vi "main.vi"() -> ()   [LabVIEW 2021]
uses:
  <vilib>/Utility/error.llb/Error Cluster From Error Code.vi
  <vilib>/ErrorRing/Error Ring.xnode
  Ctls/msg.ctl
  <vilib>/MakerHub/LINX/LMH-LINX.lvlib
  <vilib>/MakerHub/LINX/Private/Type Defs/Platform.ctl
  <vilib>/MakerHub/LINX/Private/Type Defs/Interface.ctl
  <vilib>/MakerHub/LINX/Private/Device/Type Defs/TCP Config.ctl
  <vilib>/MakerHub/LINX/Private/Device/Device.lvlib
  <vilib>/MakerHub/LINX/Private/Device/Type Defs/Channels.ctl
  <vilib>/MakerHub/LINX/Private/Device/Type Defs/LINX Device Config.ctl
  <vilib>/MakerHub/LINX/Private/Type Defs/LINX Ref.ctl
  <vilib>/MakerHub/LINX/Public/Utilities/Open Serial.vi
  Global 1.vi
panel:
  in  "Buadrate":u32=8
  out "?":bool
  out "Trama Leída w/r":string
  in  "Número de bytes a leer":u8=32
  in  "Dirección Esclavo (w/r)":u8=8
  in  "Envio":string
  in  "WaR":bool
  out "?":bool
  out "?":bool
  out "Status":bool
  in  "Stop":bool
  in  "Dirección Esclavo Escritura":u8=8
  in  "Dirección Eslcavo Lectura":u8=8
  in  "Número de bytes a leer":u8=32
  out "Trama Leída":string
  in  "Data":string
  in  "Puerto COM":refnum<visa-resource-name>
  in  "Read":bool
  in  "Write":bool
  in  "error in (no error) 3":errorcluster
  out "error in (no error) 2":errorcluster
  out "Data":u8[](array[numeric])
  in  "error in (no error)":errorcluster
  # "LECTURA"
  # "ESCRITURA"
  # "CONFIGURACIÓN"
  # "ESCRITURA/LECTURA"
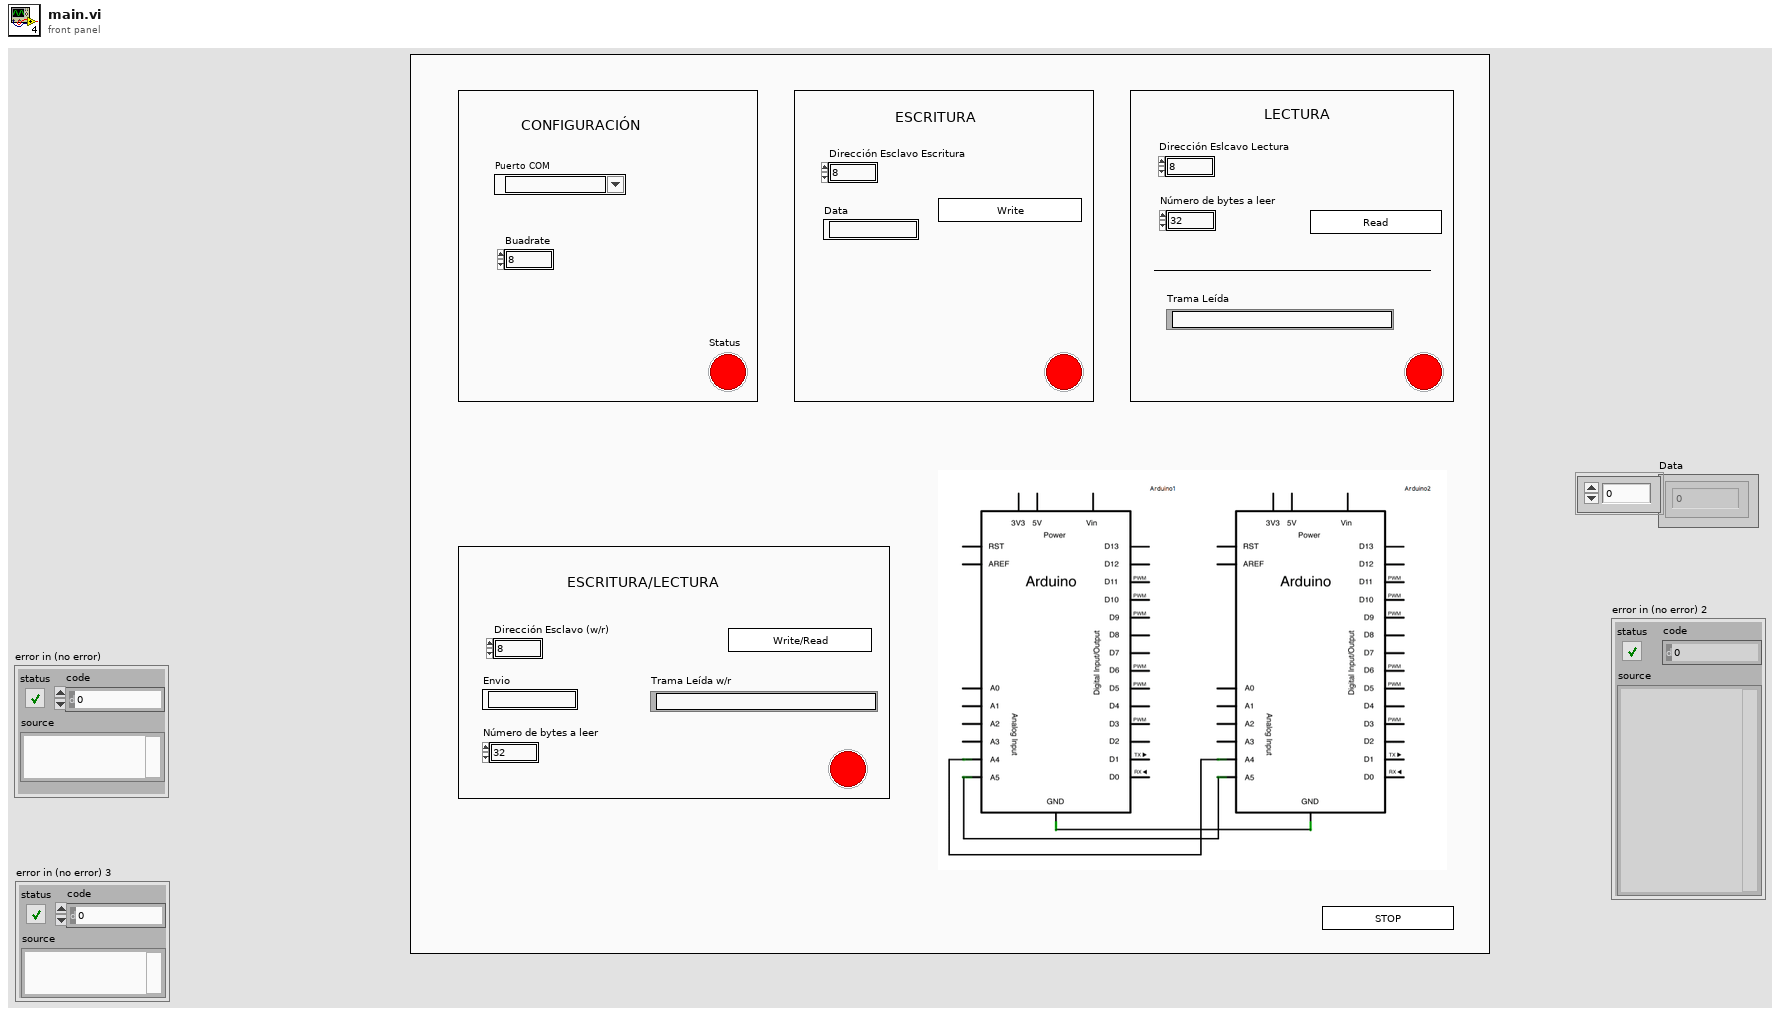
[diagram p1: front panel]
types:
  T1 = typedef "msg.ctl" = cluster{"mensaje":string, "info":cluster{"I2C Slave Address ":u8, "Data":u8[], "Bytes To Read":u8}, "LINX Resource":T2}
  T2 = typedef "LMH-LINX.lvlib/LINX Ref.ctl" = cluster{"IO":T3, "Interface":T4, "LINX Device Config":T5}
  T3 = typedef "LMH-LINX.lvlib/Platform.ctl" = enum16{"Remote", "Local"}
  T4 = typedef "LMH-LINX.lvlib/Interface.ctl" = enum16{"Serial", "TCP"}
  T5 = typedef "LMH-LINX.lvlib/Device.lvlib/LINX Device Config.ctl" = cluster{"Interface":T4, "COM Port":refnum<visa-resource-name>, "TCP Configuration":T6, "Device Family":u8, "Device ID":u8, "Device Name":string, "TCP Ref":refnum<k5>, "Channels":T7}
  T6 = typedef "LMH-LINX.lvlib/Device.lvlib/TCP Config.ctl" = cluster{"IP Address":string, "Port":u16}
  T7 = typedef "LMH-LINX.lvlib/Channels.ctl" = cluster{"DI":u8[], "DO":u8[], "AI":u8[], "AO":u8[], "PWM":u8[], "QE":u8[], "UART":u8[], "I2C 2":u8[], "SPI":u8[], "CAN":u8[], "Servo":u8[], "AI Ref (V)":dbl, "AI Resolution (Bits)":u8, "AO Ref (V)":dbl, "AO Resolution (Bits)":u8}
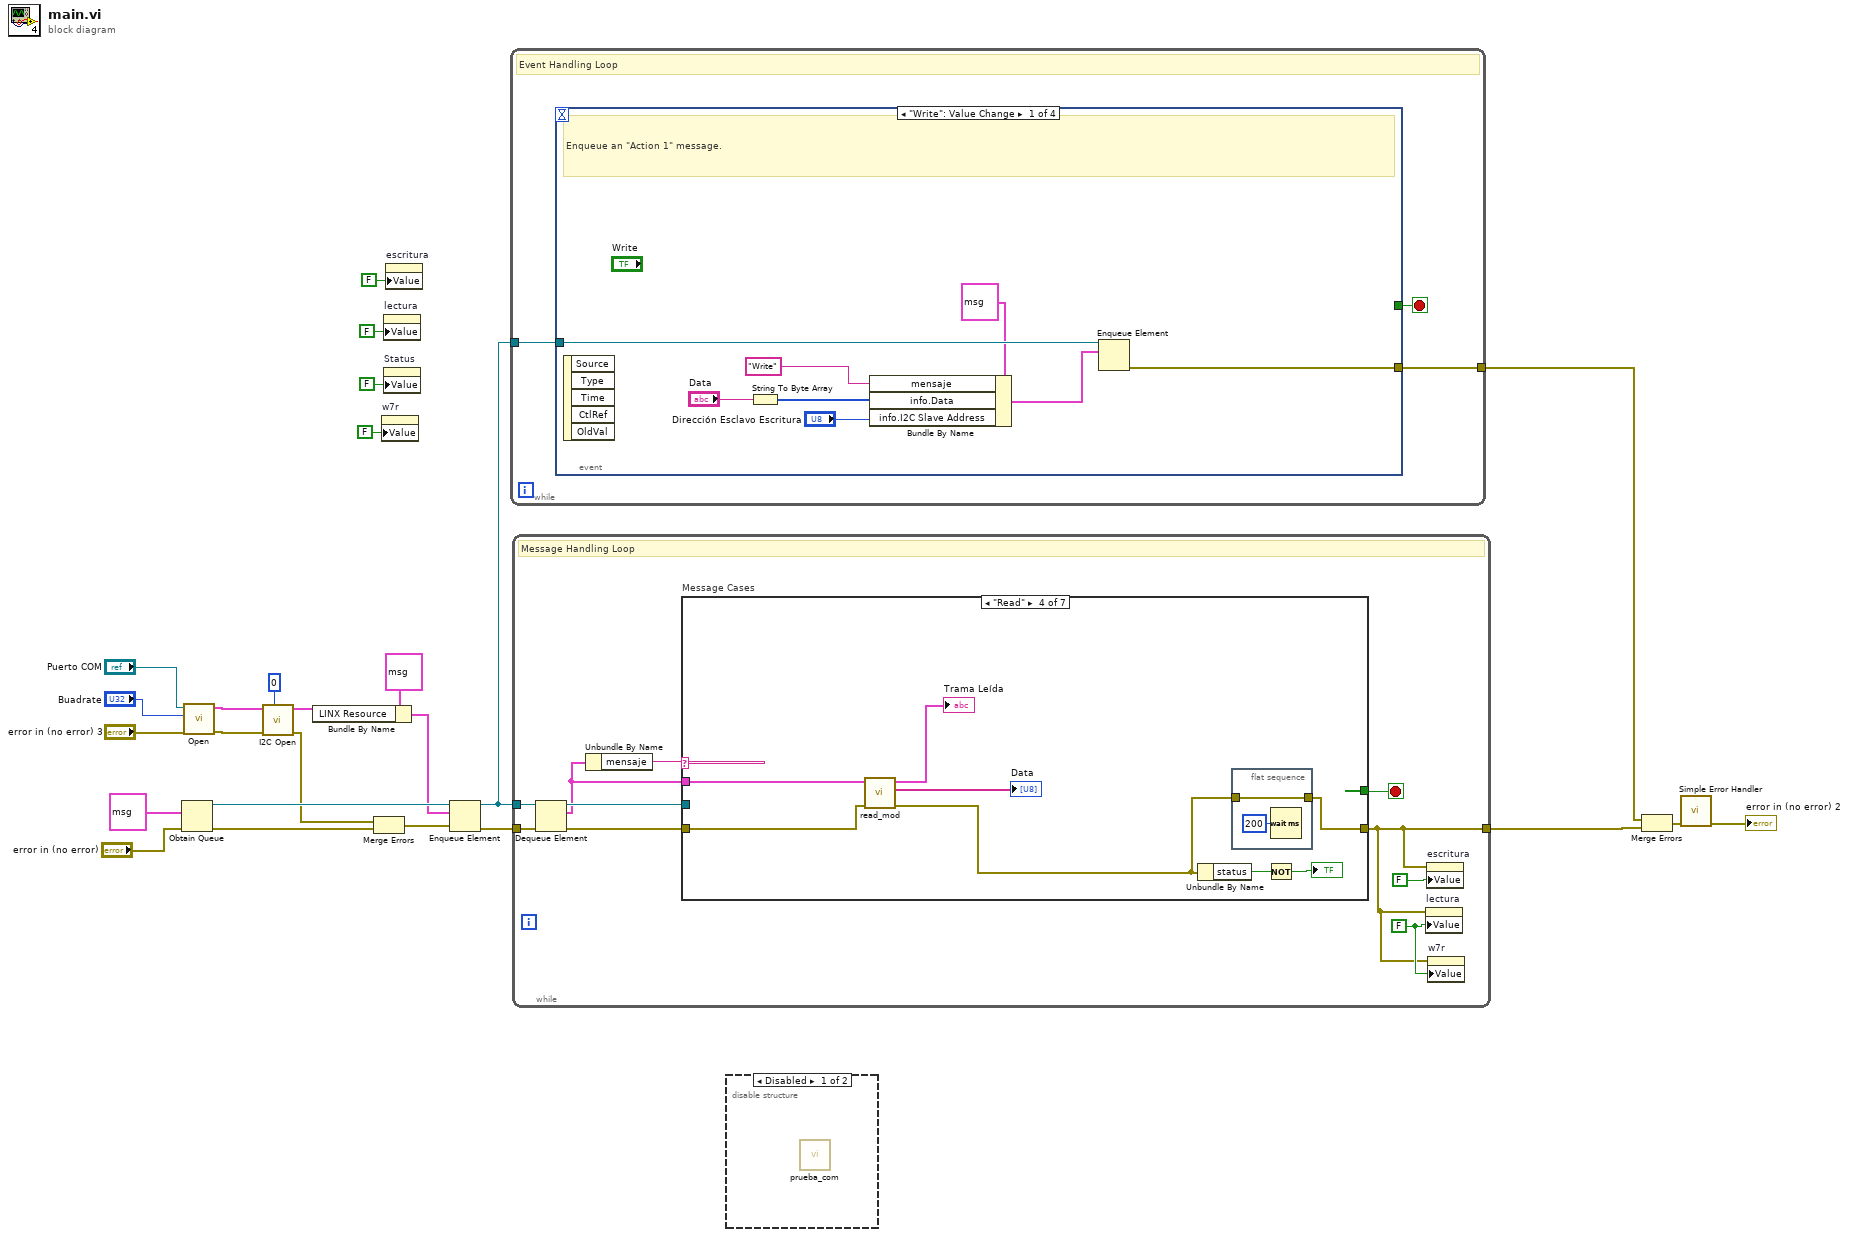
[diagram p0: block diagram]
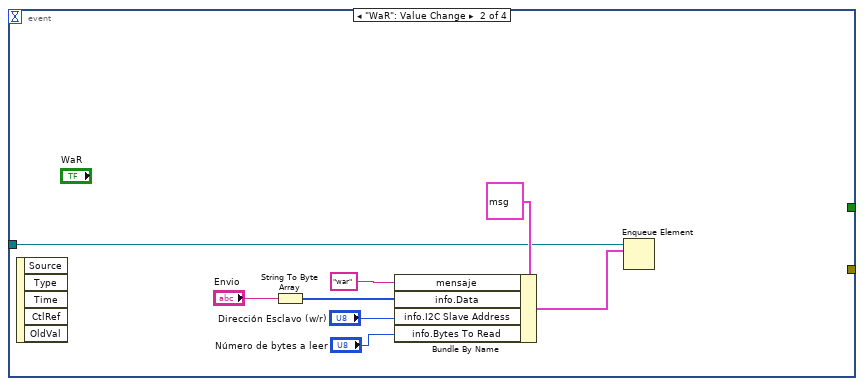
[diagram p2: hidden frame]
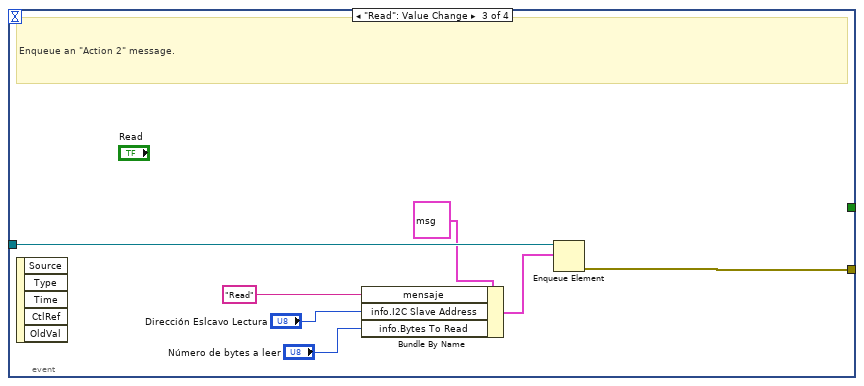
[diagram p3: hidden frame]
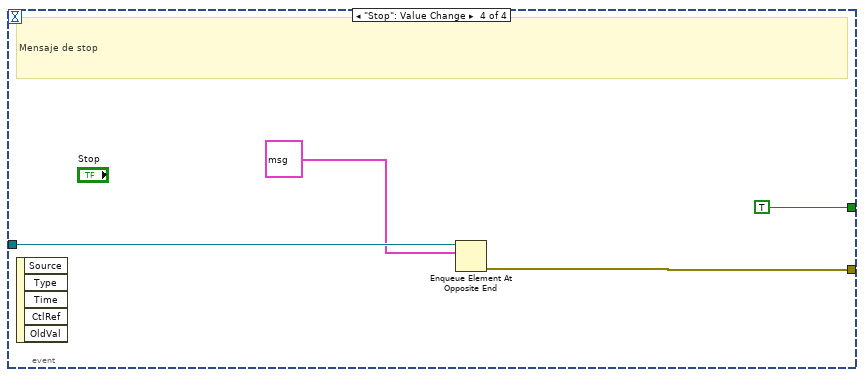
[diagram p4: hidden frame]
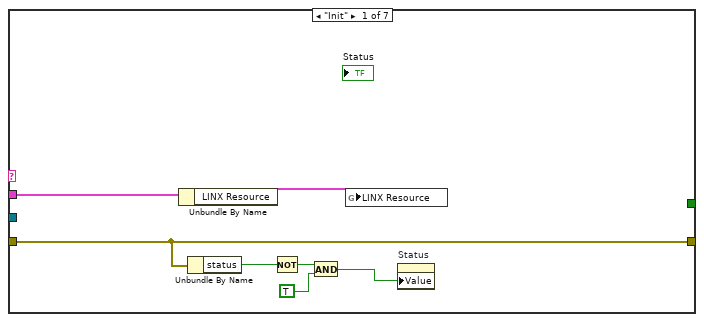
[diagram p6: hidden frame]
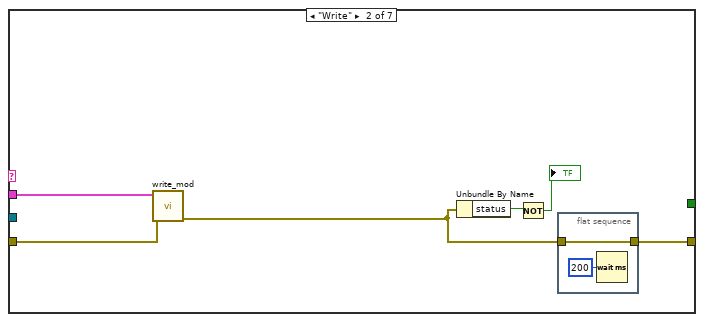
[diagram p7: hidden frame]
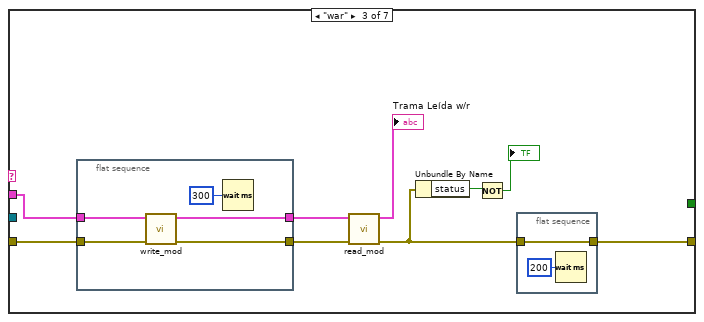
[diagram p8: hidden frame]
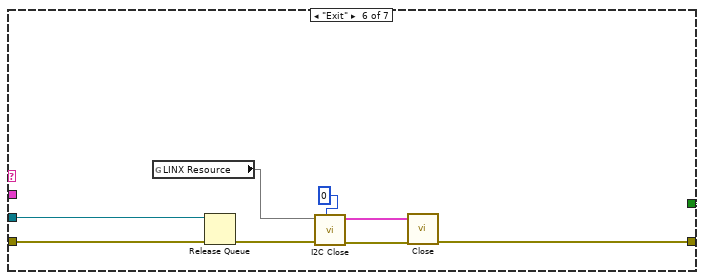
[diagram p10: hidden frame]
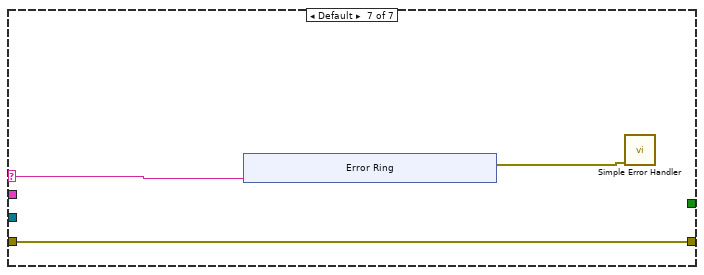
[diagram p11: hidden frame]
diagram:
  n1 = Obtain Queue(element data type=T1 {"mensaje"="Init", "info"={"I2C Slave Address "=0, "Data"=[0], "Bytes To Read"=0}, "LINX Resource"={"IO"=enum."Remote", "Interface"=enum."Serial", "LINX Device Config"={"Interface"=enum."Serial", "COM Port"="", "TCP Configuration"={"IP Address"="", "Port"=0}, "Device Family"=0, "Device ID"=0, "Device Name"="", "TCP Ref"=refnum, "Channels"={"DI"=[], "DO"=[], "AI"=[], "AO"=[], "PWM"=[], "QE"=[], "UART"=[], "I2C 2"=[], "SPI"=[], "CAN"=[], "Servo"=[], "AI Ref (V)"=0.0, "AI Resolution (Bits)"=0, "AO Ref (V)"=0.0, "AO Resolution (Bits)"=0}}}} ("msg"), error in (no error)="error in (no error)") -> (queue out=w23:refnum<queue>, error out=w17:errorcluster)  [unwired: 3 in, 1 out]
  n2 = call-poly <vilib>:"Open.vi"("Error In"="error in (no error) 3", "Baud Rate Override"="Buadrate", "Serial Port"="Puerto COM") -> ("Error Out"=w13:errorcluster, "LINX Resource"=w11:T2)  [unwired: 6 in, 1 out]
  n3 = call <vilib>:"I2C Open.vi"("I2C Channel (0)"=u8 0, "Error In"=w13, "LINX Resource"=w11) -> ("Error Out"=w9:errorcluster, "LINX Resource"=w10:T2)  [unwired: 7 in]
  n4 = Bundle By Name(cluster=T1 {"mensaje"="Init", "info"={"I2C Slave Address "=0, "Data"=[0], "Bytes To Read"=0}, "LINX Resource"={"IO"=enum."Remote", "Interface"=enum."Serial", "LINX Device Config"={"Interface"=enum."Serial", "COM Port"="", "TCP Configuration"={"IP Address"="", "Port"=0}, "Device Family"=0, "Device ID"=0, "Device Name"="", "TCP Ref"=refnum, "Channels"={"DI"=[], "DO"=[], "AI"=[], "AO"=[], "PWM"=[], "QE"=[], "UART"=[], "I2C 2"=[], "SPI"=[], "CAN"=[], "Servo"=[], "AI Ref (V)"=0.0, "AI Resolution (Bits)"=0, "AO Ref (V)"=0.0, "AO Resolution (Bits)"=0}}}} ("element 2"), "LINX Resource"=w10) -> (w14:T1)
  n5 = Merge Errors(w9, w17) -> (w16:errorcluster)
  n6 = property on="w7r" class="Bool (strict)"("Value"=FALSE) -> ()  [unwired: 2 in, 2 out]
  n7 = property on="lectura" class="Bool (strict)"("Value"=FALSE) -> ()  [unwired: 2 in, 2 out]
  n8 = property on="Status" class="Bool (strict)"("Value"=FALSE ("Status")) -> ()  [unwired: 2 in, 2 out]
  n9 = property on="escritura" class="Bool (strict)"("Value"=FALSE) -> ()  [unwired: 2 in, 2 out]
  n10 = Enqueue Element(queue=w23, element=w14, error in (no error)=w16) -> (queue out=w21:refnum<queue>, error out=w22:errorcluster)  [unwired: 1 in, 1 out]
  n11 = while {
    tunnel: w21 -> [w28]
    tunnel: [w26] -> w24
    stop <- w27 stop-if-true
    # "Event Handling Loop"
    n12 = event shown="[0] \"Write\": Value Change" {
      selector: _ -> [_ _ _ _]
      dyn-events: _ -> [_ _ _ _]
      timeout: _ -> [_ _ _ _]
      tunnel: [_ _ _ TRUE] -> w27
      tunnel: w28 -> [w34 w38 w51 w55]
      tunnel: [w36 _ w50 w54] -> w26
      event "Write": Value Change {
        # "Enqueue an \"Action 1\" message."
        n13 = event-data() -> ()  [unwired: 1 in, 5 out]
        n14 = String To Byte Array(string="Data") -> (unsigned byte array=w31:u8[])
        n15 = Bundle By Name(cluster=T1 {"mensaje"="Init", "info"={"I2C Slave Address "=0, "Data"=[0], "Bytes To Read"=0}, "LINX Resource"={"IO"=enum."Remote", "Interface"=enum."Serial", "LINX Device Config"={"Interface"=enum."Serial", "COM Port"="", "TCP Configuration"={"IP Address"="", "Port"=0}, "Device Family"=0, "Device ID"=0, "Device Name"="", "TCP Ref"=refnum, "Channels"={"DI"=[], "DO"=[], "AI"=[], "AO"=[], "PWM"=[], "QE"=[], "UART"=[], "I2C 2"=[], "SPI"=[], "CAN"=[], "Servo"=[], "AI Ref (V)"=0.0, "AI Resolution (Bits)"=0, "AO Ref (V)"=0.0, "AO Resolution (Bits)"=0}}}} ("element 2"), "mensaje"="Write", "info.Data"=w31, "info.I2C Slave Address"="Dirección Esclavo Escritura") -> (w32:T1)
        n16 = Enqueue Element(queue=w34, element=w32) -> (error out=w36:errorcluster)  [unwired: 2 in, 2 out]
      }
      event "WaR": Value Change {
        n17 = event-data() -> ()  [unwired: 1 in, 5 out]
        n18 = String To Byte Array(string="Envio") -> (unsigned byte array=w41:u8[])
        n19 = Bundle By Name(cluster=T1 {"mensaje"="Init", "info"={"I2C Slave Address "=0, "Data"=[0], "Bytes To Read"=0}, "LINX Resource"={"IO"=enum."Remote", "Interface"=enum."Serial", "LINX Device Config"={"Interface"=enum."Serial", "COM Port"="", "TCP Configuration"={"IP Address"="", "Port"=0}, "Device Family"=0, "Device ID"=0, "Device Name"="", "TCP Ref"=refnum, "Channels"={"DI"=[], "DO"=[], "AI"=[], "AO"=[], "PWM"=[], "QE"=[], "UART"=[], "I2C 2"=[], "SPI"=[], "CAN"=[], "Servo"=[], "AI Ref (V)"=0.0, "AI Resolution (Bits)"=0, "AO Ref (V)"=0.0, "AO Resolution (Bits)"=0}}}} ("element 2"), "mensaje"="war", "info.Data"=w41, "info.I2C Slave Address"="Dirección Esclavo (w/r)", "info.Bytes To Read"="Número de bytes a leer") -> (w42:T1)
        n20 = Enqueue Element(queue=w38, element=w42) -> ()  [unwired: 2 in, 3 out]
      }
      event "Read": Value Change {
        # "Enqueue an \"Action 2\" message."
        n21 = event-data() -> ()  [unwired: 1 in, 5 out]
        n22 = Bundle By Name(cluster=T1 {"mensaje"="Read", "info"={"I2C Slave Address "=0, "Data"=[0], "Bytes To Read"=0}, "LINX Resource"={"IO"=enum."Remote", "Interface"=enum."Serial", "LINX Device Config"={"Interface"=enum."Serial", "COM Port"="", "TCP Configuration"={"IP Address"="", "Port"=0}, "Device Family"=0, "Device ID"=0, "Device Name"="", "TCP Ref"=refnum, "Channels"={"DI"=[], "DO"=[], "AI"=[], "AO"=[], "PWM"=[], "QE"=[], "UART"=[], "I2C 2"=[], "SPI"=[], "CAN"=[], "Servo"=[], "AI Ref (V)"=0.0, "AI Resolution (Bits)"=0, "AO Ref (V)"=0.0, "AO Resolution (Bits)"=0}}}} ("element"), "mensaje"="Read", "info.I2C Slave Address"="Dirección Eslcavo Lectura", "info.Bytes To Read"="Número de bytes a leer") -> (w48:T1)
        n23 = Enqueue Element(queue=w51, element=w48) -> (error out=w50:errorcluster)  [unwired: 2 in, 2 out]
      }
      event "Stop": Value Change {
        # "Mensaje de stop"
        n24 = event-data() -> ()  [unwired: 1 in, 5 out]
        n25 = Enqueue Element At Opposite End(queue=w55, element=T1 {"mensaje"="Exit", "info"={"I2C Slave Address "=0, "Data"=[0], "Bytes To Read"=0}, "LINX Resource"={"IO"=enum."Remote", "Interface"=enum."Serial", "LINX Device Config"={"Interface"=enum."Serial", "COM Port"="", "TCP Configuration"={"IP Address"="", "Port"=0}, "Device Family"=0, "Device ID"=0, "Device Name"="", "TCP Ref"=refnum, "Channels"={"DI"=[], "DO"=[], "AI"=[], "AO"=[], "PWM"=[], "QE"=[], "UART"=[], "I2C 2"=[], "SPI"=[], "CAN"=[], "Servo"=[], "AI Ref (V)"=0.0, "AI Resolution (Bits)"=0, "AO Ref (V)"=0.0, "AO Resolution (Bits)"=0}}}}) -> (error out=w54:errorcluster)  [unwired: 2 in, 2 out]
      }
    }
  }
  n26 = while {
    tunnel: w21 -> [w63]
    tunnel: w22 -> [w64]
    tunnel: [w56] -> w25
    stop <- w65 stop-if-true
    w57 = FALSE
    # "Message Handling Loop"
    n27 = Dequeue Element(queue=w63, error in (no error)=w64) -> (queue out=w62:refnum<queue>, element=w59:T1, error out=w61:errorcluster)  [unwired: 1 in, 1 out]
    n28 = Unbundle By Name(w59) -> ("mensaje"=w60:string)
    n29 = case "Message Cases" shown="\"Read\"" w60 {
      selector: w60 -> [_ _ _ _ _ _ w119]
      tunnel: w62 -> [_ _ _ _ _ w116 _]
      tunnel: w61 -> [w70 w78 w89 w104 w107 w114 w118]
      tunnel: [w70 w73 w81 w98 w107 w111 w118] -> w56
      tunnel: [_ _ _ _ _ TRUE _] -> w65
      tunnel: w59 -> [w72 w77 w87 w103 _ _ _]
      frame "Init" {
        # "Initialize - Perform any initialization code for your application here. In this example, the only initialization required is setting the Display Message indicator value to an empty string."
        n30 = Unbundle By Name(w72) -> ("LINX Resource"=w71:T2)
        n31 = Unbundle By Name(w70) -> ("status"=w69:bool)
        n32 = Not(x=w69) -> (.not. x?=w68:bool)
        n33 = And(x=w68, y=TRUE ("Status")) -> (x .and. y?=w66:bool)
        n34 = global write "Global 1.vi" "LINX Resource"(w71) -> ()
        n35 = property on="Status" class="Bool (strict)"("Value"=w66) -> ()  [unwired: 2 in, 2 out]
      }
      frame "Write" {
        # "Action 1 - Send an \"Update Display\" message indicating which button was pressed. Note that a string is sent as the Message Data along with the \"Update Display\" message."
        n36 = call "write_mod.vi"("error in (no error)"=w78, 11:w77) -> ("error out"=w74:errorcluster)  [unwired: 8 in, 1 out]
        n37 = Unbundle By Name(w74) -> ("status"=w76:bool)
        n38 = Not(x=w76) -> (.not. x?=→"?":bool)
        n39 = flat-sequence {
          tunnel: w74 -> [w80]
          tunnel: [w80] -> w73
          frame #0 {
            n40 = Wait (ms)(milliseconds to wait=u32 200) -> ()  [unwired: 1 out]
          }
        }
      }
      frame "war" {
        n41 = flat-sequence {
          tunnel: w89 -> [w96]
          tunnel: [w95] -> w88
          tunnel: w87 -> [w94]
          tunnel: [w93] -> w86
          frame #0 {
            n42 = call "write_mod.vi"("error in (no error)"=w96, 11:w94) -> ("error out"=w95:errorcluster, "msg 3"=w93:T1)  [unwired: 8 in]
            n43 = Wait (ms)(milliseconds to wait=u32 300) -> ()  [unwired: 1 out]
          }
        }
        n44 = call "read_mod.vi"("error in (no error)"=w88, "msg"=w86) -> ("error out"=w82:errorcluster, "output cluster"=→"Trama Leída w/r":T1)  [unwired: 6 in, 2 out]
        n45 = Unbundle By Name(w82) -> ("status"=w84:bool)
        n46 = Not(x=w84) -> (.not. x?=→"?":bool)
        n47 = flat-sequence {
          tunnel: w82 -> [w91]
          tunnel: [w91] -> w81
          frame #0 {
            n48 = Wait (ms)(milliseconds to wait=u32 200) -> ()  [unwired: 1 out]
          }
        }
      }
      frame "Read" {
        # "sdff"
        n49 = call "read_mod.vi"("error in (no error)"=w104, "msg"=w103) -> ("error out"=w99:errorcluster, "Datos Leídos"=→"Data":string[], "output cluster"=→"Trama Leída":T1)  [unwired: 6 in, 1 out]
        n50 = Unbundle By Name(w99) -> ("status"=w101:bool)
        n51 = flat-sequence {
          tunnel: w99 -> [w106]
          tunnel: [w106] -> w98
          frame #0 {
            n52 = Wait (ms)(milliseconds to wait=u32 200) -> ()  [unwired: 1 out]
          }
        }
        n53 = Not(x=w101) -> (.not. x?=→"?":bool)
      }
      frame "Update Display" {
        # "Update Display - Convert the Message Data to a string to display in the Display Message indicator."
      }
      frame "Exit" {
        # "Exit - Exit the application. Since this message was sent as a priority message (i.e., it was placed at the front of the queue), any cleanup code should run here, since the loop is about to stop. Any other messages in the queue will not be handled."
        n54 = global read "Global 1.vi" "LINX Resource"() -> (w109)
        n55 = Release Queue(queue=w116, error in (no error)=w114) -> (error out=w113:errorcluster)  [unwired: 1 in, 2 out]
        n56 = call <vilib>:"I2C Close.vi"("I2C Channel (0)"=u8 0, "Error In"=w113, "LINX Resource"=w109) -> ("Error Out"=w112:errorcluster, "LINX Resource"=w108:T2)  [unwired: 7 in]
        n57 = call <vilib>:"Close.vi"("Error In"=w112, "LINX Resource"=w108) -> ("Error Out"=w111:errorcluster)  [unwired: 9 in]
      }
      frame Default {
        # "The Default case only runs if there is a message that isn't defined in any of the other cases. Generate an error if this occurs."
        n58 = xnode "Error Ring"("parameter 0"=w119) -> ("error out"=w117:errorcluster)
        n59 = call <vilib>:"Simple Error Handler.vi"("error in (no error)"=w117) -> ()  [unwired: 4 in, 5 out]
      }
    }
    n60 = property on="lectura" class="Bool (strict)"(error in=w56, "Value"=w57) -> ()  [unwired: 1 in, 2 out]
    n61 = property on="escritura" class="Bool (strict)"(error in=w56, "Value"=FALSE) -> ()  [unwired: 1 in, 2 out]
    n62 = property on="w7r" class="Bool (strict)"(error in=w56, "Value"=w57) -> ()  [unwired: 1 in, 2 out]
  }
  n63 = disable-structure shown="Disabled" {
    frame Disabled {
      n64 = call "prueba_com.vi"() -> ()  [unwired: 12 in]
    }
    frame Enabled {
    }
  }
  n65 = Merge Errors(w24, w25) -> (w20:errorcluster)
  n66 = call <vilib>:"Simple Error Handler.vi"("error in (no error)"=w20) -> ("error out"=→"error in (no error) 2":errorcluster)  [unwired: 4 in, 4 out]
